vi "Fix_YAML.vi"(11 "Array in":string[](array[string])) -> (3 "Array out":string[](array[string]))   [LabVIEW 2016]
uses:
  <userlib>/_OpenG.lib/dictionary/dictionary.llb/Dictionary Key Value Pair Cluster__ogtk.ctl
  <userlib>/_OpenG.lib/dictionary/dictionary.llb/Dictionary Update (by scalar value)__ogtk.vi
panel:
  out "created new?":bool
  out "String":string
  out "substring before match":string
  out "error out":errorcluster
  in  "error in (no error)":errorcluster
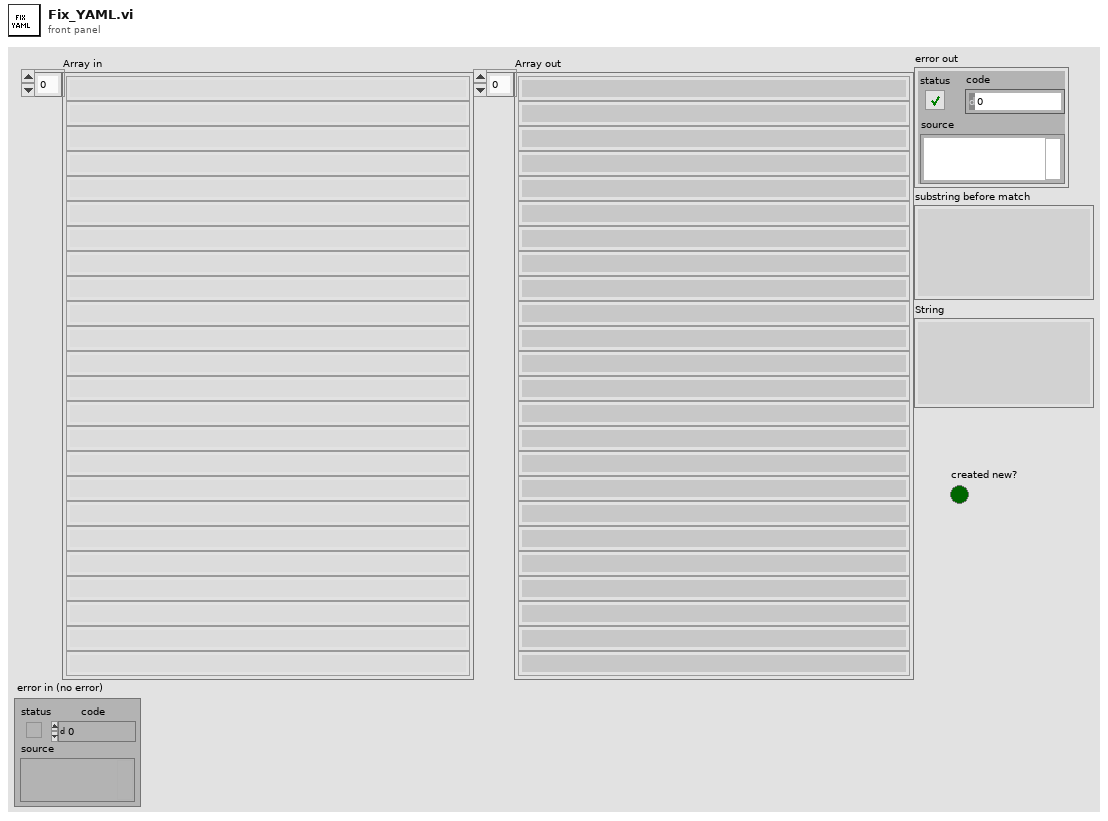
[diagram p1: front panel]
types:
  T1 = typedef "Dictionary Object RefNum__ogtk.ctl" = refnum<k1>
  T2 = typedef "Dictionary Key Value Pair Cluster__ogtk.ctl" = cluster{"key":variant, "value":variant}
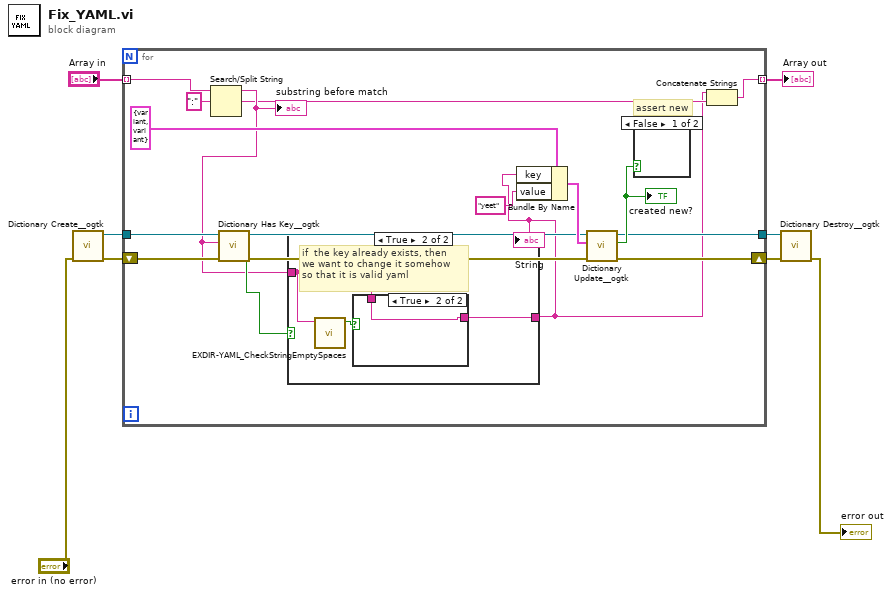
[diagram p0: block diagram]
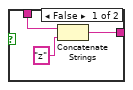
[diagram p4: hidden frame]
diagram:
  n1 = call <userlib>:"Dictionary Create__ogtk.vi"("error in (no error)"="error in (no error)") -> ("error out"=w6:errorcluster, "dictionary out"=w4:T1)  [unwired: 9 in]
  n2 = for {
    tunnel: "Array in" -> [w10] mode=indexing
    tunnel: [w9] -> w8 mode=indexing
    shift-right: [w14] -> w2
    shift-left: w6 -> [w20]
    tunnel: w4 -> [w21]
    tunnel: [w13] -> w3
    # "assert new"
    n3 = Search/Split String(string=w10, search string/char (-)=":") -> (substring before match=w18:string, match + rest of string=w12:string)  [unwired: 1 in, 1 out]
    "substring before match" <- w18
    n4 = call <userlib>:"Dictionary Has Key__ogtk.vi"("error in (no error)"=w20, "key"=w18, "dictionary"=w21) -> ("error out"=w15:errorcluster, "Has Key?"=w19:bool, "dictionary out"=w16:T1)  [unwired: 6 in]
    n5 = case shown="True" w19 {
      tunnel: w18 -> [w26 w28]
      tunnel: [w26 w29] -> w11
      frame False {
        # "if it doesn't exist,\nadd it as is"
      }
      frame True {
        # "if  the key already exists, then\nwe want to change it somehow\nso that it is valid yaml"
        n6 = call "EXDIR-YAML_CheckStringEmptySpaces.vi"("String"=w28) -> ("empty or all spaces"=w27:bool)  [unwired: 10 in]
        n7 = case shown="True" w27 {
          tunnel: [w31 w33] -> w29
          tunnel: w28 -> [w30 w33]
          frame False {
            n8 = Concatenate Strings(w30, "z") -> (w31:string)
          }
          frame True {
          }
        }
      }
    }
    "String" <- w11
    n9 = Bundle By Name(cluster=T2 {"key"=variant, "value"=variant} ("key-value"), "key"=w11, "value"="yeet") -> (w22:T2)
    n10 = call-poly <userlib>:"Dictionary Update__ogtk.vi"("error in (no error)"=w15, "key-value"=w22, "dictionary"=w16) -> ("error out"=w14:errorcluster, "created new?"=w17:bool, "dictionary out"=w13:T1)  [unwired: 6 in]
    "created new?" <- w17
    n11 = case shown="False" w17 {
      frame False {
      }
      frame True {
      }
    }
    n12 = Concatenate Strings(w11, w12) -> (w9:string)
  }
  "Array out" <- w8
  n13 = call <userlib>:"Dictionary Destroy__ogtk.vi"("error in (no error)"=w2, "dictionary"=w3) -> ("error out"=→"error out":errorcluster)  [unwired: 9 in]
